vi "BLEMISH_DETECT.vi"(0 "Range (Image [Threshold])":cluster{"Lower value":sgl, "Upper value":sgl}={"Lower value"=167.0, "Upper value"=255.0}, 1 "Min Radius (Circle Detection)":sgl=20.0, 2 "Max Radius (Circle Detection)":sgl=500.0, 7 "error in":errorcluster, 8 "File Path":path=path "C:/SNAPSHOT.bmp") -> (20 "Nb Circles (Circle Detection)":i32, 21 "Circles Data (Circle Detection)":T3(array[cluster]), 22 "ROI Pixel Statistics (Line Profile)":T2 {"Min" format="%.2f"; "Std Dev" format="%.2f"; "Mean" format="%.2f"; "Max" format="%.2f"}, 23 "Percent Contrast":sgl, 24 "Diameter":i32, 27 "error out":errorcluster)   [LabVIEW 2014]
uses:
  <vilib>/vision/NI_Vision_Development_Module.lvlib
panel:
  out "Image Out":T1(plugin-control)
  out "Line Profile Graph":cluster{"x0":sgl, "dx":sgl, "Pixels Line":sgl[]}(graph) caption="Line Profile"
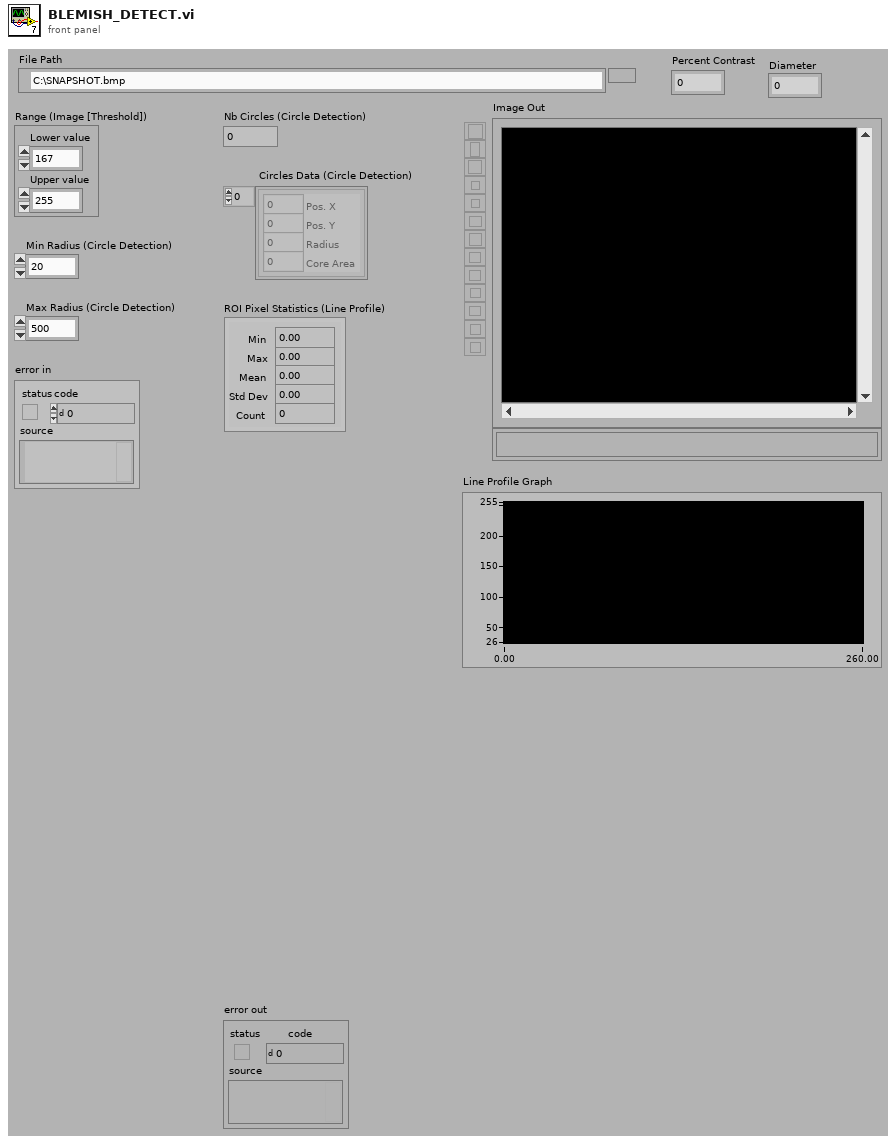
[diagram p1: front panel]
types:
  T1 = typedef "IMAQ Image.ctl" = refnum<image>
  T2 = cluster{"Min":sgl, "Max":sgl, "Mean":sgl, "Std Dev":sgl, "Count":i32}
  T3 = cluster{"Pos. X":i32, "Pos. Y":i32, "Radius":i32, "Core Area":i32}[]
  T4 = cluster{"Global Rectangle":i32[], "Contours":cluster{"ID":enum32{"External", "Internal"}, "Type":u32, "Coordinates":i32[]}[]}
  T5 = cluster{"Origin":cluster{"X":sgl, "Y":sgl}, "Angle (deg)":sgl, "Axis Reference":u32}
  T6 = enum16{"Reset", "Update Coordinate System", "Get Coordinate System"}
  T7 = enum16{"Horizontal Motion", "Vertical Motion", "Horizontal and Vertical Motion", "Horizontal, Vertical and Angular Motion"}
  T8 = typedef "Image Type" = u32
  T9 = cluster{"Circles Data[0]":cluster{"Pos. X":i32, "Pos. Y":i32, "Radius":i32, "Core Area":i32}, "Circles Data[1]":cluster{"Pos. X":i32, "Pos. Y":i32, "Radius":i32, "Core Area":i32}, "Circles Data[2]":cluster{"Pos. X":i32, "Pos. Y":i32, "Radius":i32, "Core Area":i32}, "Circles Data[3]":cluster{"Pos. X":i32, "Pos. Y":i32, "Radius":i32, "Core Area":i32}, "Circles Data[4]":cluster{"Pos. X":i32, "Pos. Y":i32, "Radius":i32, "Core Area":i32}, "Circles Data[5]":cluster{"Pos. X":i32, "Pos. Y":i32, "Radius":i32, "Core Area":i32}, "Circles Data[6]":cluster{"Pos. X":i32, "Pos. Y":i32, "Radius":i32, "Core Area":i32}, "Circles Data[7]":cluster{"Pos. X":i32, "Pos. Y":i32, "Radius":i32, "Core Area":i32}, "Circles Data[8]":cluster{"Pos. X":i32, "Pos. Y":i32, "Radius":i32, "Core Area":i32}}
  T10 = typedef "IMAQ Coordinate System" = cluster{"Reference System":cluster{"Origin":cluster{"X":sgl, "Y":sgl}, "Angle (deg)":sgl, "Axis Reference":u32}, "Measurement System":cluster{"Origin":cluster{"X":sgl, "Y":sgl}, "Angle (deg)":sgl, "Axis Reference":u32}}
  T11 = typedef "ROI Descriptor" = cluster{"Global Rectangle":i32[], "Contours":cluster{"ID":enum32{"External", "Internal"}, "Type":u32, "Coordinates":i32[]}[]}
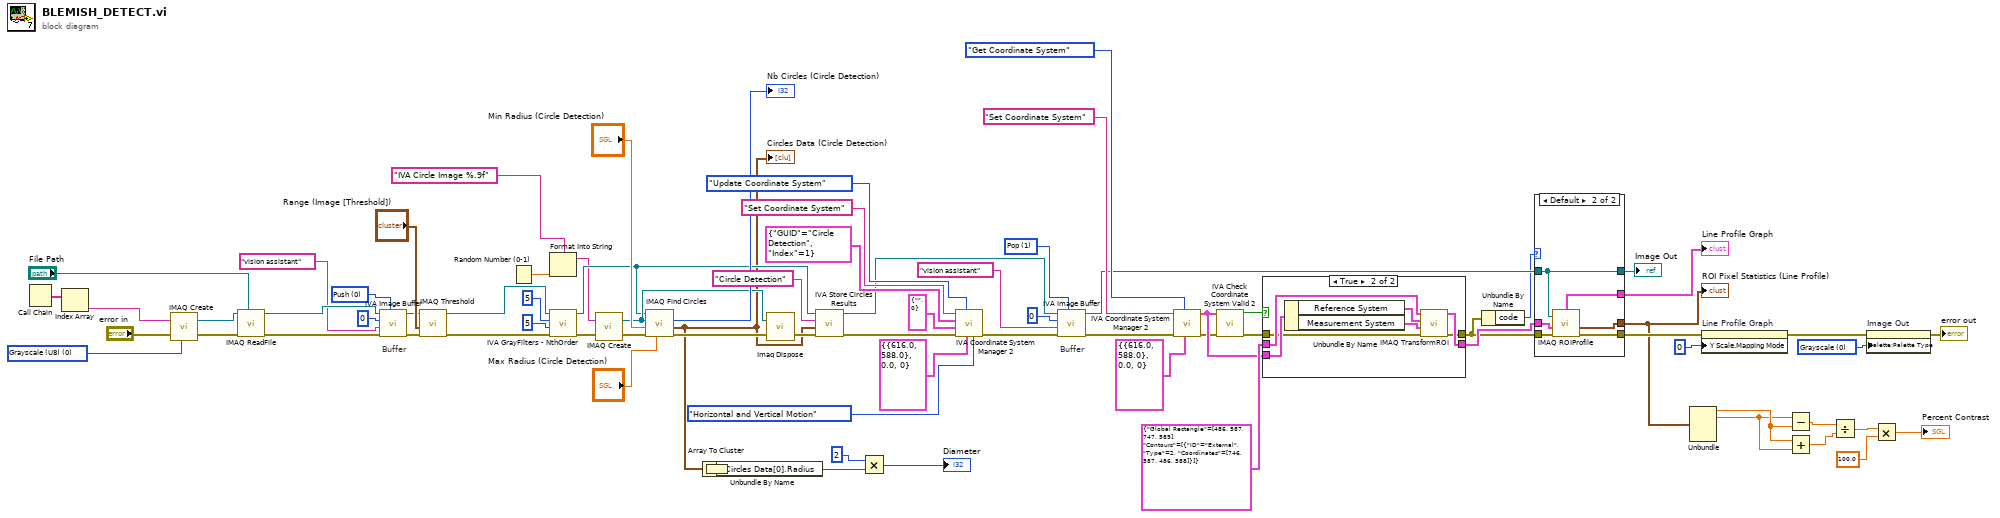
[diagram p0: block diagram]
diagram:
  w17 = u32 0 items=["Grayscale", "Binary", "Gradient", "Rainbow", "Temperature", "User Defined"] ("Palette")
  w37 = u16 1 items=["Push", "Pop", "Reset"] ("Function")
  w69 = u16 0 items=["Push", "Pop", "Reset"] ("Function")
  w72 = T8 0 items=["Grayscale (U8)", "Grayscale (I16)", "Grayscale (SGL)", "Complex (CSG)", "RGB (U32)", "HSL (U32)", "RGB (U64)", "Grayscale (U16)"] ("Image Type")
  # "Buffer"
  # "Buffer"
  n1 = Call Chain() -> (call chain=w74:string[])
  n2 = Index Array(array=w74) -> (element=w73:string)  [unwired: 1 in]
  n3 = call "IMAQ Create"("Image Name"=w73, "Image Type"=w72, "error in (no error)"="error in") -> ("New Image"=w77:T1, "error out"=w76:errorcluster)  [unwired: 1 in, 1 out]
  n4 = call "IMAQ ReadFile"("File Path"="File Path", "error in (no error)"=w76, "Image"=w77) -> ("error out"=w70:errorcluster, "Image Out"=w71:T1)  [unwired: 2 in, 5 out]
  n5 = call <vilib>:"IVA Image Buffer.vi"("Function"=w69, "error in (no error)"=w70, "Prefix"="vision assistant", "Buffer #"=0, "Image In"=w71) -> ("error out"=w64:errorcluster, "Image Out"=w65:T1)  [unwired: 5 out]
  n6 = call "IMAQ Threshold"("error in (no error)"=w64, "Range"="Range (Image [Threshold])", "Image Src"=w65) -> ("error out"=w62:errorcluster, "Image Dst Out"=w63:T1)  [unwired: 3 in, 4 out]
  n7 = Random Number (0-1)() -> (number: 0 to 1=w47:dbl)
  n8 = Format Into String(format string="IVA Circle Image %.9f" ("Image Name"), w47) -> (resulting string=w49:string)  [unwired: 2 in, 1 out]
  n9 = call <vilib>:"IVA GrayFilters - NthOrder.vi"("error in"=w62, "Filter size Y"=5, "Filter size X"=5, "Image In"=w63) -> ("error out"=w54:errorcluster, "Image Out"=w51:T1)  [unwired: 6 out]
  n10 = call "IMAQ Create"("Image Name"=w49, "error in (no error)"=w54) -> ("New Image"=w56:T1, "error out"=w55:errorcluster)  [unwired: 2 in, 1 out]
  n11 = call "IMAQ Find Circles"("Max Radius"="Max Radius (Circle Detection)", "error in (no error)"=w55, "Min Radius"="Min Radius (Circle Detection)", "Image Dst"=w56, "Image Src"=w51) -> ("error out"=w53:errorcluster, "Circles Data"=w3:T3, "Nb Circles"=→"Nb Circles (Circle Detection)":i32)  [unwired: 4 out]
  "Circles Data (Circle Detection)" <- w3
  n12 = Array To Cluster(array=w3) -> (cluster=w7:T9)
  n13 = Unbundle By Name(w7) -> ("Circles Data[0].Radius"=w6:i32)
  n14 = call "Imaq Dispose"("Image"=w56, "error in (no error)"=w53) -> ("error out"=w52:errorcluster)  [unwired: 1 in, 3 out]
  n15 = call <vilib>:"IVA Store Circles Results.vi"("error in (no error)"=w52, "Circles Data"=w3, "Step Name"="Circle Detection", "Image in"=w51) -> ("error out"=w40:errorcluster, "Image dup"=w39:T1)  [unwired: 6 out]
  n16 = Multiply(x=2, y=w6) -> (x*y=→"Diameter":i32)
  n17 = call <vilib>:"IVA Coordinate System Manager 2.vi"("Mode"=T7."Horizontal and Vertical Motion", "Reference System"=T5 {"Origin"={"X"=616.0, "Y"=588.0}, "Angle (deg)"=0.0, "Axis Reference"=0}, "Function"=T6."Update Coordinate System", "error in (no error)"=w40, "Angle ID"=cluster{"GUID":string, "Index":i32} {"GUID"="", "Index"=0}, "Origin ID"=cluster{"GUID":string, "Index":i32} {"GUID"="Circle Detection", "Index"=1}, "Coordinate System Name"="Set Coordinate System") -> ("error out"=w38:errorcluster)  [unwired: 4 out]
  n18 = call <vilib>:"IVA Image Buffer.vi"("Function"=w37, "error in (no error)"=w38, "Prefix"="vision assistant", "Buffer #"=0, "Image In"=w39) -> ("error out"=w32:errorcluster, "Image Out"=w23:T1)  [unwired: 5 out]
  n19 = call <vilib>:"IVA Coordinate System Manager 2.vi"("Reference System"=T5 {"Origin"={"X"=616.0, "Y"=588.0}, "Angle (deg)"=0.0, "Axis Reference"=0}, "Function"=T6."Get Coordinate System", "error in (no error)"=w32, "Coordinate System Name"="Set Coordinate System") -> ("error out"=w27:errorcluster, "Coordinate System Out"=w29:T10)  [unwired: 3 in, 3 out]
  n20 = call <vilib>:"IVA Check Coordinate System Valid 2.vi"("error in (no error)"=w27, "Coordinate System"=w29) -> ("error out"=w26:errorcluster, "Valid?"=w28:bool)  [unwired: 8 out]
  n21 = case shown="True" w28 {
    tunnel: T4 {"Global Rectangle"=[486, 587, 747, 589], "Contours"=[{"ID"=enum."External", "Type"=2, "Coordinates"=[746, 587, 486, 588]}]} ("ROI Descriptor") -> [w79 w86]
    tunnel: [w79 w83] -> w21
    tunnel: [w78 w82] -> w20
    tunnel: w29 -> [_ w81]
    tunnel: w26 -> [w78 w80]
    frame False {
    }
    frame True {
      n22 = Unbundle By Name(w81) -> ("Reference System"=w85:T5, "Measurement System"=w84:T5)
      n23 = call "IMAQ TransformROI"("error in (no error)"=w80, "New Reference"=w84, "Base Reference"=w85, "ROI Descriptor"=w86) -> ("error out"=w82:errorcluster, "ROI Descriptor out"=w83:T11)  [unwired: 6 out]
    }
  }
  n24 = Unbundle By Name(w20) -> ("code"=w19:i32)
  n25 = case shown="Default" w19 {
    tunnel: w20 -> [_ w93]
    tunnel: [_ w92] -> w9
    tunnel: [_ w91] -> w24
    tunnel: w23 -> [w87 w88]
    tunnel: [_ w90] -> w22
    tunnel: w21 -> [_ w89]
    tunnel: [w87 w88] -> w18
    frame -1074396199, -1074396198 {
      # "Discard\nCoordinate\nSystem\nError"
    }
    frame Default {
      n26 = call "IMAQ ROIProfile"("error in (no error)"=w93, "ROI Descriptor"=w89, "Image"=w88) -> ("ROI Pixel Statistics"=w92:T2, "error out"=w91:errorcluster, "ROI Graph"=w90:cluster{"x0":sgl, "dx":sgl, "Pixels Line":sgl[]})  [unwired: 3 out]
    }
  }
  "ROI Pixel Statistics (Line Profile)" <- w9
  "Line Profile Graph" <- w22
  "Image Out" <- w18
  n27 = Unbundle(w9) -> ("Min"=w13:sgl, "Max"=w12:sgl)  [unwired: 3 out]
  n28 = property on="Line Profile Graph" class="WFGraph (strict)"(error in=w24, "Y Scale.Mapping Mode"=u8 0) -> (error out=w16:errorcluster)  [unwired: 1 in, 1 out]
  n29 = Subtract(x=w12, y=w13) -> (x-y=w11:sgl)
  n30 = Add(x=w13, y=w12) -> (x+y=w10:sgl)
  n31 = Divide(x=w11, y=w10) -> (x/y=w8:sgl)
  n32 = property on="Image Out" class="ImageControl"(error in=w16, "Palette:Palette Type"=w17) -> (error out=→"error out":errorcluster)  [unwired: 1 in, 1 out]
  n33 = Multiply(x=w8, y=sgl 100.0) -> (x*y=→"Percent Contrast":sgl)
